vi "pressurama-labview.vi"() -> ()   [LabVIEW 2021]
uses:
  <vilib>/Instr/_visa.llb/VISA Configure Serial Port (Instr).vi
panel:
  out "Freq":dbl
  in  "VISA resource name":refnum<visa-resource-name>="COM5"
  out "Waveform Chart":cluster{dbl, dbl, dbl, dbl, dbl, dbl, dbl, dbl}(graph)={17.4, 17.3, 17.4, 17.5, 17.7, 17.6, 17.5, 17.3}
  out "x = y?":bool=TRUE
  out "trimmed string":string="0:17.40 1:17.30 2:17.40 3:17.50 4:17.70 5:17.60 6:17.50 7:17.30"
  out "number of replacements":i32=7
  in  "stop":bool
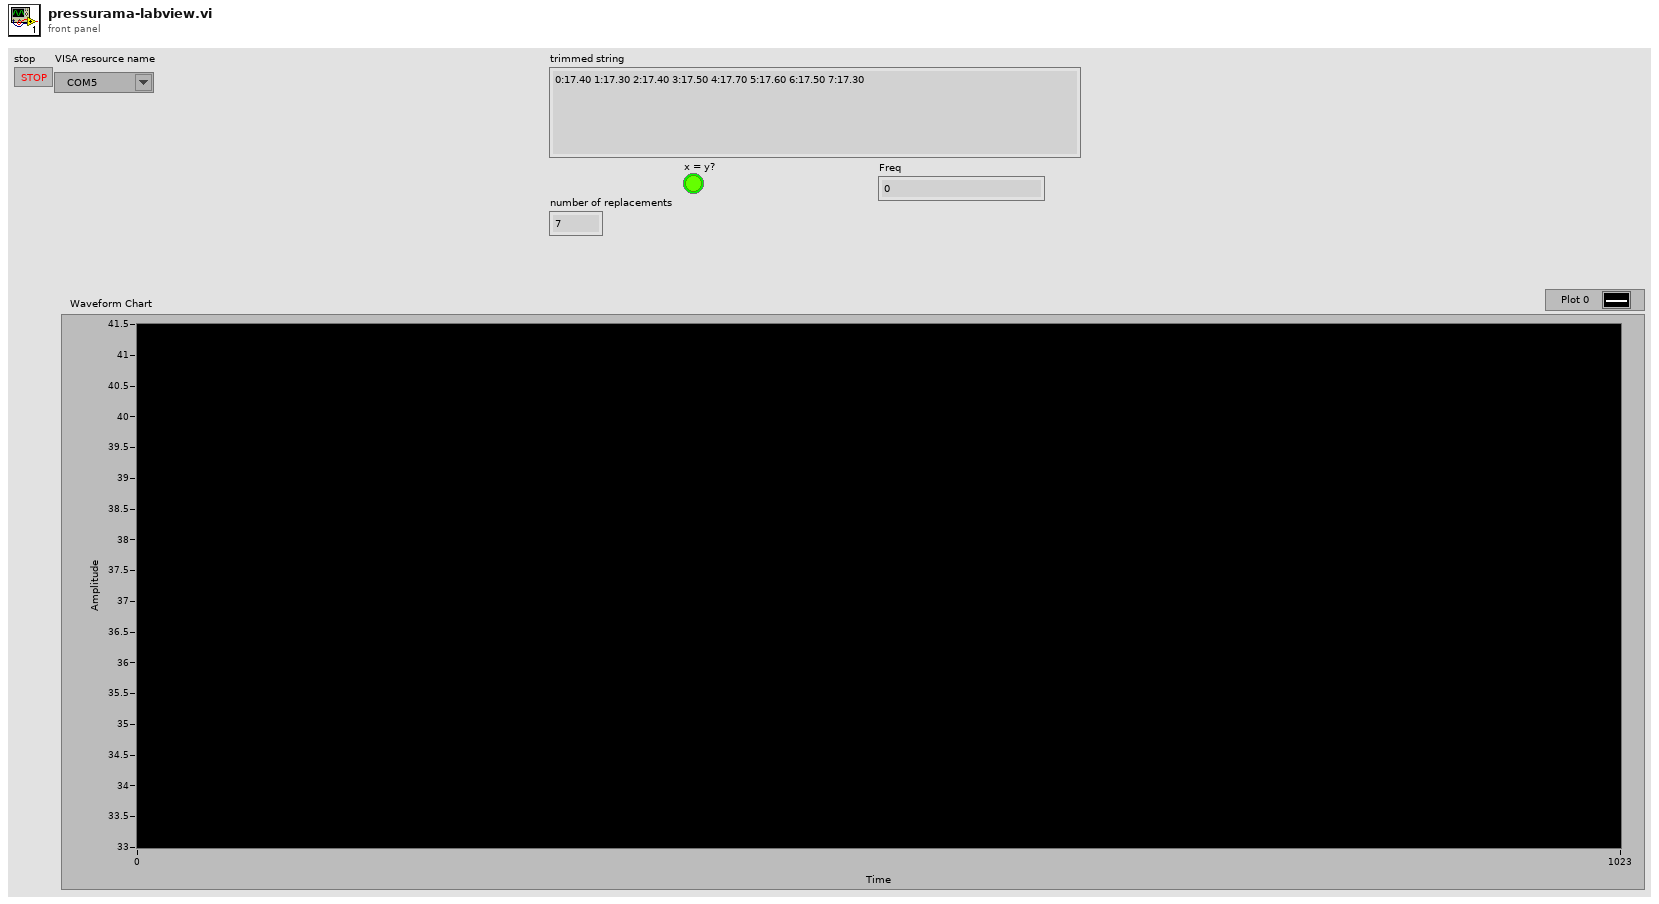
[diagram p1: front panel]
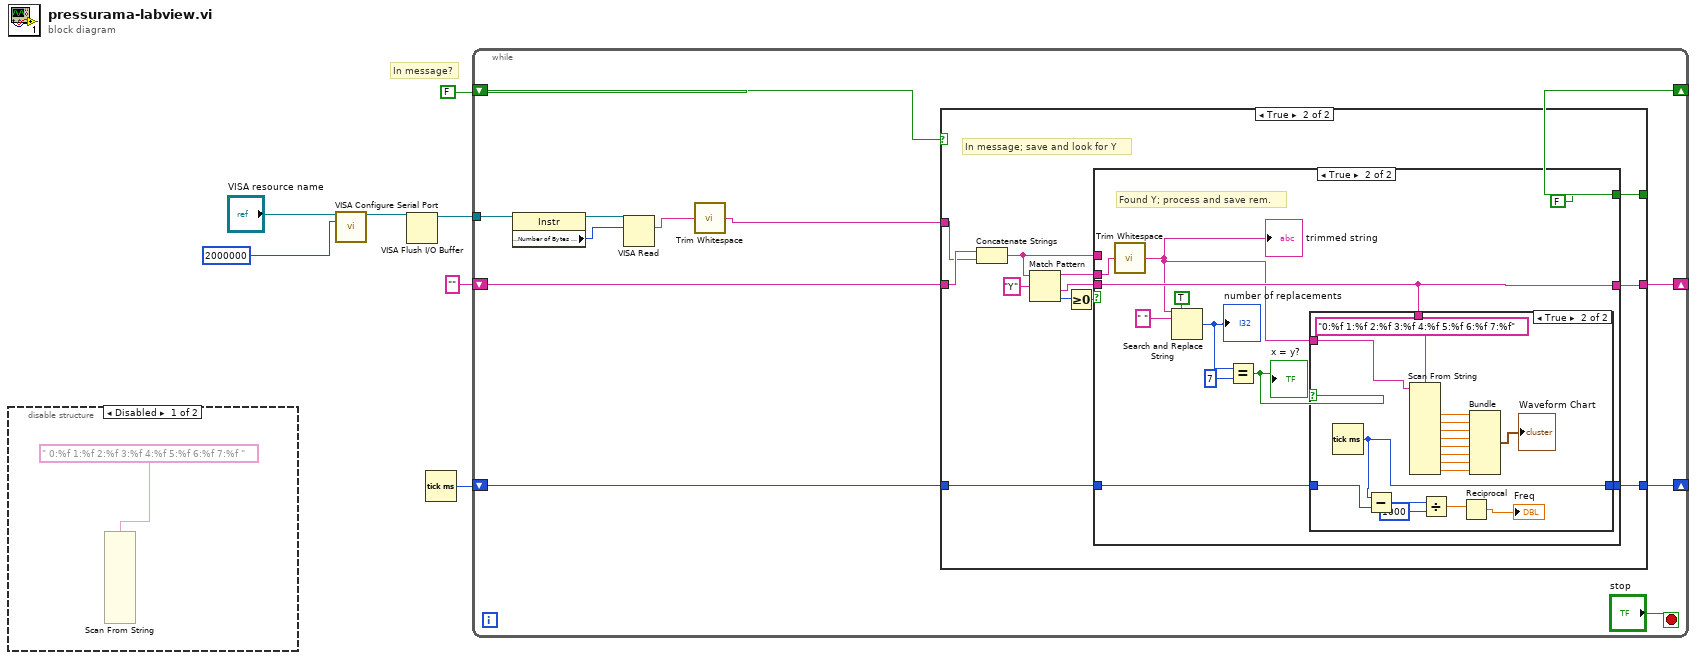
[diagram p0: block diagram]
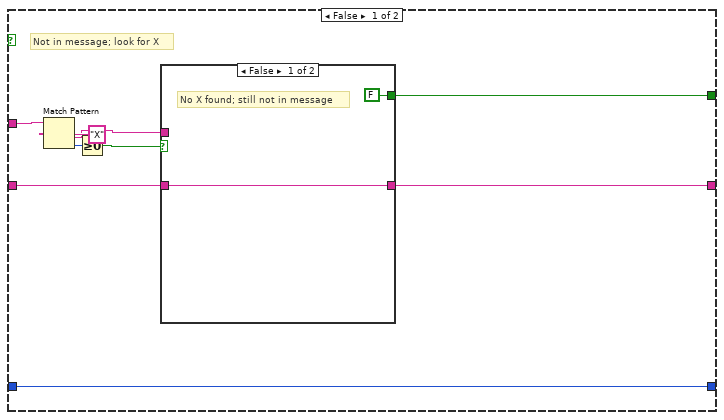
[diagram p3: hidden frame]
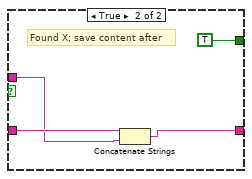
[diagram p4: hidden frame]
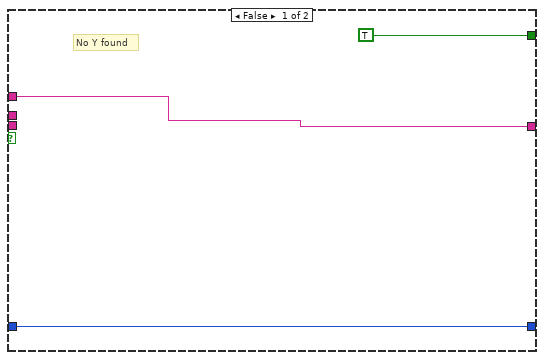
[diagram p5: hidden frame]
diagram:
  # "In message?"
  n1 = disable-structure shown="Disabled" {
    frame Disabled {
      n2 = Scan From String(format string=" 0:%f 1:%f 2:%f 3:%f 4:%f 5:%f 6:%f 7:%f ") -> ()  [unwired: 19 in, 3 out]
    }
    frame Enabled {
    }
  }
  n3 = call-poly "VISA Configure Serial Port"("VISA resource name"="VISA resource name", "baud rate (9600)"=u32 2000000) -> ("VISA resource name out"=w6:refnum<visa-resource-name>)  [unwired: 12 in, 1 out]
  n4 = VISA Flush I/O Buffer(VISA resource name=w6) -> (VISA resource name out=w5:refnum<visa-resource-name>)  [unwired: 2 in, 1 out]
  n5 = Tick Count (ms)() -> (millisecond timer value=w1:u32)
  n6 = while {
    tunnel: w5 -> [w19]
    shift-right: [w13] -> _
    shift-left: "" -> [w15]
    shift-right: [w14] -> _
    shift-left: FALSE -> [w16]
    shift-right: [w9] -> _
    shift-left: w1 -> [w10]
    stop <- "stop" stop-if-true
    n7 = property class="Instr"(reference=w19) -> (reference out=w18:refnum<visa-resource-name>, "Serial Settings:Number of Bytes at Serial Port"=w17:u32)  [unwired: 1 in, 1 out]
    n8 = VISA Read(VISA resource name=w18, byte count=w17) -> (read buffer=w12:string)  [unwired: 1 in, 3 out]
    n9 = call <vilib>:"Trim Whitespace.vi"("string"=w12) -> ("trimmed string"=w11:string)  [unwired: 1 in]
    n10 = case shown="True" w16 {
      tunnel: w11 -> [w29 w46]
      tunnel: w15 -> [w24 w47]
      tunnel: [w23 w38] -> w14
      tunnel: [w22 w40] -> w13
      tunnel: w10 -> [w21 w37]
      tunnel: [w21 w36] -> w9
      frame False {
        # "Not in message; look for X"
        n11 = Match Pattern(string=w29, regular expression="X") -> (after substring=w25:string, offset past match=w27:i32)  [unwired: 1 in, 2 out]
        n12 = Greater Or Equal To 0?(x=w27) -> (x >= 0?=w26:bool)
        n13 = case shown="False" w26 {
          tunnel: w25 -> [_ w34]
          tunnel: w24 -> [w30 w35]
          tunnel: [FALSE TRUE] -> w23
          tunnel: [w30 w32] -> w22
          frame False {
            # "No X found; still not in message"
          }
          frame True {
            # "Found X; save content after"
            n14 = Concatenate Strings(w35, w34) -> (w32:string)
          }
        }
      }
      frame True {
        # "In message; save and look for Y"
        n15 = Concatenate Strings(w47, w46) -> (w39:string)
        n16 = Match Pattern(string=w39, regular expression="Y") -> (before substring=w42:string, after substring=w41:string, offset past match=w45:i32)  [unwired: 1 in, 1 out]
        n17 = Greater Or Equal To 0?(x=w45) -> (x >= 0?=w43:bool)
        n18 = case shown="True" w43 {
          tunnel: w42 -> [_ w59]
          tunnel: [w50 w54] -> w40
          tunnel: w41 -> [_ w54]
          tunnel: w39 -> [w50 _]
          tunnel: [TRUE FALSE] -> w38
          tunnel: w37 -> [w48 w52]
          tunnel: [w48 w51] -> w36
          frame False {
            # "No Y found"
          }
          frame True {
            # "Found Y; process and save rem."
            n19 = call <vilib>:"Trim Whitespace.vi"("string"=w59) -> ("trimmed string"=w53:string)  [unwired: 1 in]
            "trimmed string" <- w53
            n20 = Search and Replace String(replace all?=TRUE ("replace all? (F)"), input string=w53, search string=" ") -> (number of replacements=w57:i32)  [unwired: 5 in, 3 out]
            "number of replacements" <- w57
            n21 = Equal?(x=w57, y=7) -> (x = y?=w55:bool)
            "x = y?" <- w55
            n22 = case shown="True" w55 {
              tunnel: w54 -> [_ _]
              tunnel: w53 -> [_ w78]
              tunnel: w52 -> [w62 w67]
              tunnel: [w62 w68] -> w51
              frame False {
              }
              frame True {
                n23 = Tick Count (ms)() -> (millisecond timer value=w68:u32)
                n24 = Subtract(x=w68, y=w67) -> (x-y=w65:u32)
                n25 = Scan From String(format string="0:%f 1:%f 2:%f 3:%f 4:%f 5:%f 6:%f 7:%f", input string=w78) -> (output 1=w77:dbl, output 2=w70:dbl, output 3=w71:dbl, output 4=w72:dbl, output 5=w73:dbl, output 6=w74:dbl, output 7=w75:dbl, output 8=w76:dbl)  [unwired: 10 in, 3 out]
                n26 = Divide(x=w65, y=u32 1000) -> (x/y=w63:dbl)
                n27 = Reciprocal(x=w63) -> (1/x=→"Freq":dbl)
                n28 = Bundle(w77, w70, w71, w72, w73, w74, w75, w76) -> (→"Waveform Chart":cluster{dbl, dbl, dbl, dbl, dbl, dbl, dbl, dbl})  [unwired: 1 in]
              }
            }
          }
        }
      }
    }
  }
